vi "Battery_Model_Continuous_Current.vi"() -> ()   [LabVIEW 2015]
uses:
  <vilib>/Platform/TimedLoop/XDataNode/timing_clust.ctl
  <vilib>/Platform/TimedLoop/XDataNode/nitl_modes.ctl
  <vilib>/Platform/TimedLoop/XDataNode/wakeup.ctl
  Global 1.vi
  <vilib>/platform/TimedLoop/XDataNode/XDataNode.xnode
  <vilib>/Utility/NIReport.llb/NI_report.lvclass
  <instrlib>/Agilent N6700 Series/Agilent N6700 Series.lvlib
  <vilib>/Platform/TimedLoop/XDataNode/XDNodeRunTimeDep.lvlib
  <vilib>/addons/_office/NI_ReportGenerationToolkit.lvlib
panel:
  in  "Stop":bool
  out "Voltage Graph":dbl[](graph)
  in  "Negative Voltage Limit (0.0 volts) 3":dbl format="%^.3e"
  in  "Priority (1: Voltage) 3":i32(ring) items=["Voltage"=1, "Current"=0]
  in  "Positive Voltage Limit  (5.0 V) 3":dbl=5.0 format="%^.3e"
  in  "Channel Name (1) 3":string="4"
  in  "VISA resource name 3":refnum<visa-resource-name>="USB0::0x0957::0x0F07::MY53002228::INSTR"
  in  "report file path 4":path=path "C:/Users/Tulio/Documents/LabView Projects/Battery Model/Battery_Model_Measurements.xlsx"
  out "Current Graph":dbl[](graph)
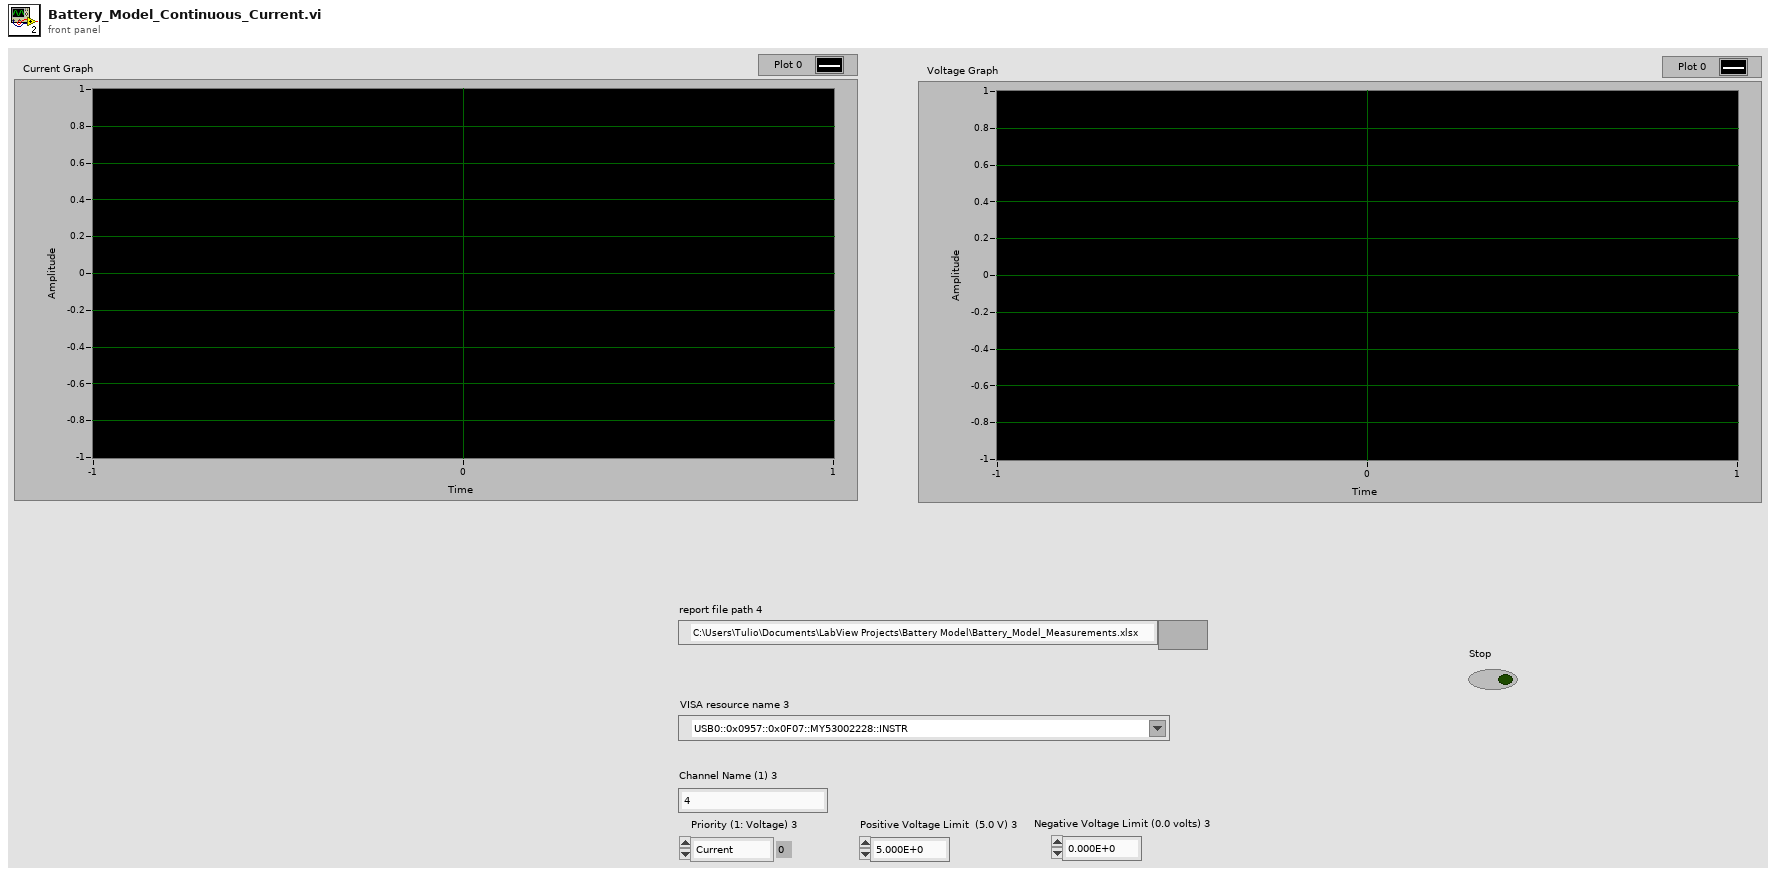
[diagram p1: front panel]
types:
  T1 = enum16{"Standard Report", "HTML", "Word", "Excel"}
  T2 = typedef "XDNodeRunTimeDep.lvlib/timing_clust.ctl" = cluster{"Expected End [f-1]":u64, "Actual End [f-1]":u64, "Finished Late? [f-1]":bool, "Expected End [i-1]":u64, "Actual End [i-1]":u64, "Finished Late? [i-1]":bool, "Expected Start [i]":u64, "Actual Start [i]":u64, "Expected Start [f]":u64, "Actual Start [f]":u64, "Source Name":string, "Structure Name":string, "Period":i64, "Deadline":i64, "Offset":i64, "Start":i64, "Priority":i32, "Timeout":i32, "Mode":T3, "Wakeup Reason":T4, "Error":errorcluster, "Source Type":string, "Secondary Source Type":string, "Global End Time":u64, "Global Start Time":u64, "Frame Duration":u64, "Iteration Duration":u64, "Assigned CPU":i32, "I/O Scan Engine Mode":u32}
  T3 = typedef "XDNodeRunTimeDep.lvlib/nitl_modes.ctl" = enum32{"No Change", "Process missed periods, maintain original phase", "Discard missed periods, maintain original phase", "Process missed periods, ignore original phase", "Discard missed periods, ignore original phase"}
  T4 = typedef "XDNodeRunTimeDep.lvlib/wakeup.ctl" = enum32{"Normal", "Aborted", "Asynchronous wakeup", "Timing source error", "Timed loop error", "Timeout"}
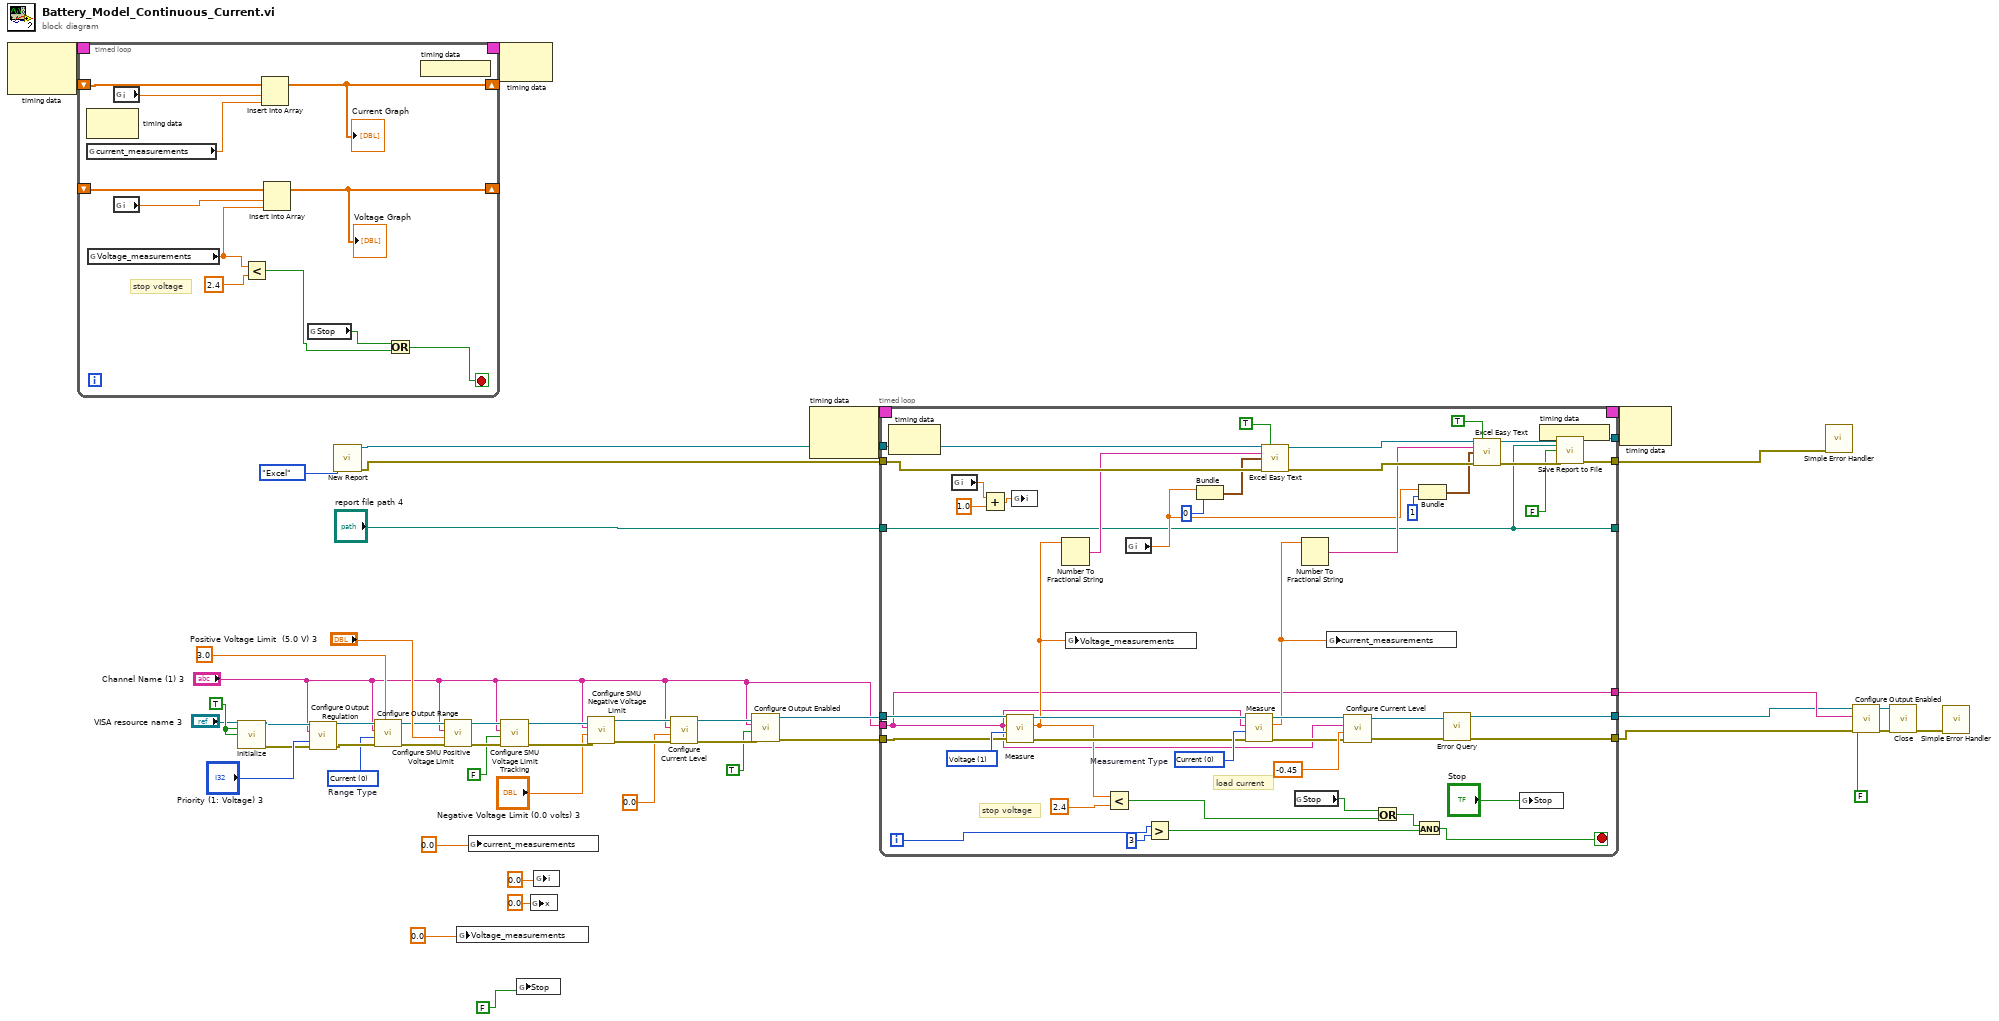
[diagram p0: block diagram]
diagram:
  w35 = TRUE ("Reset? (T: Yes)")
  w34 = 0 items=["Voltage"=1, "Current"=0]  # Range Type
  n1 = node-c288() -> (w48:T2)  [unwired: 2 in]
  n2 = timed-loop {
    timing: w48 -> [_]
    timing-out: [_] -> w47
    shift-right: [w59] -> _
    shift-left: _ -> [w60]
    shift-right: [w55] -> _
    shift-left: _ -> [w54]
    stop <- w52 stop-if-true
    # "stop voltage"
    n3 = node-c288() -> ()  [unwired: 1 in, 1 out]
    n4 = global read "Global 1.vi" "current_measurements"() -> (w57:dbl)
    n5 = global read "Global 1.vi" "Voltage_measurements"() -> (w51:dbl)
    n6 = global read "Global 1.vi" "i"() -> (w58:dbl)
    n7 = global read "Global 1.vi" "i"() -> (w56:dbl)
    n8 = Less?(x=w51, y=2.4) -> (x < y?=w50:bool)
    n9 = Insert Into Array(array=w60, index=w58, new element=w57) -> (w59:dbl[])
    "Current Graph" <- w59
    n10 = Insert Into Array(array=w54, index=w56, new element=w51) -> (w55:dbl[])
    "Voltage Graph" <- w55
    n11 = global read "Global 1.vi" "Stop"() -> (w53:bool)
    n12 = Or(x=w53, y=w50) -> (x .or. y?=w52:bool)
    n13 = node-c288() -> ()  [unwired: 1 out]
  }
  n14 = call <instrlib>:"Initialize.vi"("VISA resource name"="VISA resource name 3", "ID Query? (T: Yes)"=w35, "Reset? (T: Yes)"=w35) -> ("VISA resource name out"=w24:refnum<visa-resource-name>, "error out"=w23:errorcluster)  [unwired: 11 in]
  n15 = call <instrlib>:"Configure Output Regulation.vi"("VISA resource name"=w24, "Channel Name (1)"="Channel Name (1) 3", "Output Regulation Priority (1: Voltage)"="Priority (1: Voltage) 3", "error in (no error)"=w23) -> ("VISA resource name out"=w36:refnum<visa-resource-name>, "error out"=w37:errorcluster)  [unwired: 10 in]
  n16 = call <vilib>:"New Report.vi"("report type"=T1."Excel") -> ("report out"=w10:refnum<class "NI_report.lvclass">, "error out"=w9:errorcluster)  [unwired: 13 in]
  n17 = call <instrlib>:"Configure Output Range.vi"("Range (0.0)"=3.0, "error in (no error)"=w37, "Range Type (1: Voltage)"=w34, "Channel Name (1)"="Channel Name (1) 3", "VISA resource name"=w36) -> ("error out"=w39:errorcluster, "VISA resource name out"=w38:refnum<visa-resource-name>)  [unwired: 5 in]
  n18 = call <instrlib>:"Configure SMU Positive Voltage Limit.vi"("error in (no error)"=w39, "Positive Voltage Limit (0.0 volts)"="Positive Voltage Limit  (5.0 V) 3", "Channel Name (1)"="Channel Name (1) 3", "VISA resource name"=w38) -> ("error out"=w41:errorcluster, "VISA resource name out"=w40:refnum<visa-resource-name>)  [unwired: 6 in]
  n19 = global write "Global 1.vi" "Voltage_measurements"(0.0 ("Actual_hour")) -> ()
  n20 = global write "Global 1.vi" "current_measurements"(0.0 ("Actual_hour")) -> ()
  n21 = node-c288(w47) -> ()  [unwired: 1 out]
  n22 = call <instrlib>:"Configure SMU Voltage Limit Tracking.vi"("error in (no error)"=w41, "Enable Voltage Limit Tracking (False)"=FALSE, "Channel Name (1)"="Channel Name (1) 3", "VISA resource name"=w40) -> ("error out"=w28:errorcluster, "VISA resource name out"=w29:refnum<visa-resource-name>)  [unwired: 6 in]
  n23 = global write "Global 1.vi" "Stop"(FALSE ("Stop")) -> ()
  n24 = global write "Global 1.vi" "x"(0.0 ("x")) -> ()
  n25 = global write "Global 1.vi" "i"(0.0 ("Actual_hour")) -> ()
  n26 = call <instrlib>:"Configure SMU Negative Voltage Limit.vi"("error in (no error)"=w28, "Negative Voltage Limit (0.0 volts)"="Negative Voltage Limit (0.0 volts) 3", "Channel Name (1)"="Channel Name (1) 3", "VISA resource name"=w29) -> ("error out"=w25:errorcluster, "VISA resource name out"=w26:refnum<visa-resource-name>)  [unwired: 6 in]
  n27 = call <instrlib>:"Configure Current Level.vi"("error in (no error)"=w25, "Level  (0.0 A)"=0.0, "Channel Name (1)"="Channel Name (1) 3", "VISA resource name"=w26) -> ("error out"=w44:errorcluster, "VISA resource name out"=w45:refnum<visa-resource-name>)  [unwired: 6 in]
  n28 = call <instrlib>:"Configure Output Enabled.vi"("error in (no error)"=w44, "Enable Output (False)"=TRUE, "Channel Name (1)"="Channel Name (1) 3", "VISA resource name"=w45) -> ("error out"=w6:errorcluster, "VISA resource name out"=w7:refnum<visa-resource-name>)  [unwired: 6 in]
  n29 = node-c288() -> (w12:T2)  [unwired: 2 in]
  n30 = timed-loop {
    timing: w12 -> [_]
    timing-out: [_] -> w11
    tunnel: w10 -> [w108]
    tunnel: "Channel Name (1) 3" -> [w64]
    tunnel: [w76] -> _
    tunnel: "report file path 4" -> [w70]
    tunnel: w7 -> [w92]
    tunnel: [w87] -> w2
    tunnel: [w86] -> w4
    tunnel: w9 -> [w107]
    tunnel: [w96] -> w1
    tunnel: w6 -> [w71]
    tunnel: [w70] -> _
    tunnel: [w64] -> w3
    i -> [w68]
    stop <- w66 stop-if-true
    w91 = 1 items=["Current", "Voltage", "Power"] ("Measurement Type (1: Voltage)")
    w109 = 0 items=["Voltage"=1, "Current"=0]  # Measurement Type
    # "stop voltage"
    # "load current"
    n31 = node-c288() -> ()  [unwired: 1 in, 1 out]
    n32 = global read "Global 1.vi" "i"() -> (w80:dbl)
    n33 = Add(x=w80, y=1.0) -> (x+y=w81:dbl)
    n34 = call <instrlib>:"Measure.vi"("error in (no error)"=w71, "Measurement Type (1: Voltage)"=w91, "Channel Name (1)"=w64, "VISA resource name"=w92) -> ("error out"=w94:errorcluster, "Measurement"=w74:dbl, "VISA resource name out"=w93:refnum<visa-resource-name>)  [unwired: 5 in]
    n35 = global write "Global 1.vi" "i"(w81) -> ()
    n36 = Number To Fractional String(number=w74) -> (F-format string=w90:string)  [unwired: 3 in]
    n37 = global write "Global 1.vi" "Voltage_measurements"(w74) -> ()
    n38 = Less?(x=w74, y=2.4) -> (x < y?=w73:bool)
    n39 = global read "Global 1.vi" "i"() -> (w78:dbl)
    n40 = Greater?(x=w68, y=3) -> (0:w65:bool)
    n41 = Bundle("i"=w78, "offset (0)"=0) -> (w106:cluster{"i":dbl, "offset (0)":i32})  [unwired: 1 in]
    n42 = call <instrlib>:"Measure.vi"("error in (no error)"=w94, "Measurement Type (1: Voltage)"=w109, "Channel Name (1)"=w64, "VISA resource name"=w93) -> ("error out"=w82:errorcluster, "Measurement"=w77:dbl, "VISA resource name out"=w83:refnum<visa-resource-name>)  [unwired: 5 in]
    n43 = call <vilib>:"Excel Easy Text.vi"("report in"=w108, "border? (F)"=TRUE, "text"=w90, "start (-1, -1)"=w106, "error in (no error)"=w107) -> ("report out"=w103:refnum<class "NI_report.lvclass">, "error out"=w104:errorcluster)  [unwired: 6 in, 3 out]
    n44 = global read "Global 1.vi" "Stop"() -> (w75:bool)
    n45 = Number To Fractional String(number=w77) -> (F-format string=w100:string)  [unwired: 3 in]
    n46 = global write "Global 1.vi" "current_measurements"(w77) -> ()
    n47 = call <instrlib>:"Configure Current Level.vi"("error in (no error)"=w82, "Level  (0.0 A)"=-0.45, "Channel Name (1)"=w64, "VISA resource name"=w83) -> ("error out"=w84:errorcluster, "VISA resource name out"=w85:refnum<visa-resource-name>)  [unwired: 6 in]
    n48 = Or(x=w75, y=w73) -> (x .or. y?=w67:bool)
    n49 = And(x=w67, y=w65) -> (x .and. y?=w66:bool)
    n50 = Bundle("i"=w78, "offset (0)"=1) -> (w101:cluster{"i":dbl, "offset (0)":i32})  [unwired: 1 in]
    n51 = call <instrlib>:"Error Query.vi"("VISA resource name"=w85, "error in (no error)"=w84) -> ("VISA resource name out"=w87:refnum<visa-resource-name>, "error out"=w86:errorcluster)  [unwired: 10 in, 2 out]
    n52 = call <vilib>:"Excel Easy Text.vi"("report in"=w103, "border? (F)"=TRUE, "text"=w100, "start (-1, -1)"=w101, "error in (no error)"=w104) -> ("report out"=w98:refnum<class "NI_report.lvclass">, "error out"=w97:errorcluster)  [unwired: 6 in, 3 out]
    n53 = global write "Global 1.vi" "Stop"("Stop") -> ()
    n54 = node-c288() -> ()  [unwired: 1 out]
    n55 = call-dynamic "Save Report to File.vi"("report in"=w98, "report file path"=w70, "prompt to replace? (F)"=FALSE, "error in (no error)"=w97) -> ("report out"=w76:refnum<class "NI_report.lvclass">, "error out"=w96:errorcluster)  [unwired: 10 in]
  }
  n56 = node-c288(w11) -> ()  [unwired: 1 out]
  n57 = call <vilib>:"Simple Error Handler.vi"("error in (no error)"=w1) -> ()  [unwired: 1 in, 8 out]
  n58 = call <instrlib>:"Configure Output Enabled.vi"("error in (no error)"=w4, "Enable Output (False)"=FALSE, "Channel Name (1)"=w3, "VISA resource name"=w2) -> ("error out"=w15:errorcluster, "VISA resource name out"=w14:refnum<visa-resource-name>)  [unwired: 6 in]
  n59 = call <instrlib>:"Close.vi"("VISA resource name"=w14, "error in (no error)"=w15) -> ("error out"=w13:errorcluster)  [unwired: 13 in]
  n60 = call <vilib>:"Simple Error Handler.vi"("error in (no error)"=w13) -> ()  [unwired: 4 in, 5 out]
